vi "Ordering System.vi"() -> ()   [LabVIEW 2022 SP3]
panel:
  out "Waiting time":i32
  in  "Place your order":bool
  out "Discount %":string
  out "Discounted Bill":dbl
  out "Bill":dbl
  out "Price 5":dbl
  in  "Quantity":dbl=1.0 min=1.0 max=10.0 step=1.0
  in  "Item #1 5":bool
  out "Price 4":dbl
  in  "Quantity":dbl=1.0 min=1.0 max=10.0 step=1.0
  in  "Item #4":bool
  out "Price 3":dbl
  in  "Quantity":dbl=1.0 min=1.0 max=10.0 step=1.0
  in  "Item #3":bool
  out "Price 2":dbl
  in  "Quantity":dbl=1.0 min=1.0 max=10.0 step=1.0
  in  "Item #2":bool
  out "Price":dbl
  in  "Quantity":dbl=1.0 min=1.0 max=10.0 step=1.0
  in  "Item #1":bool
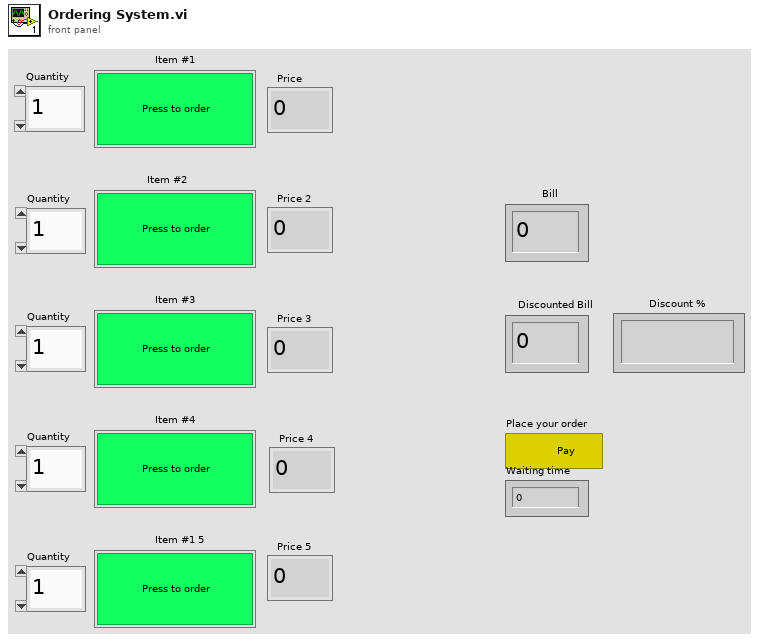
[diagram p1: front panel]
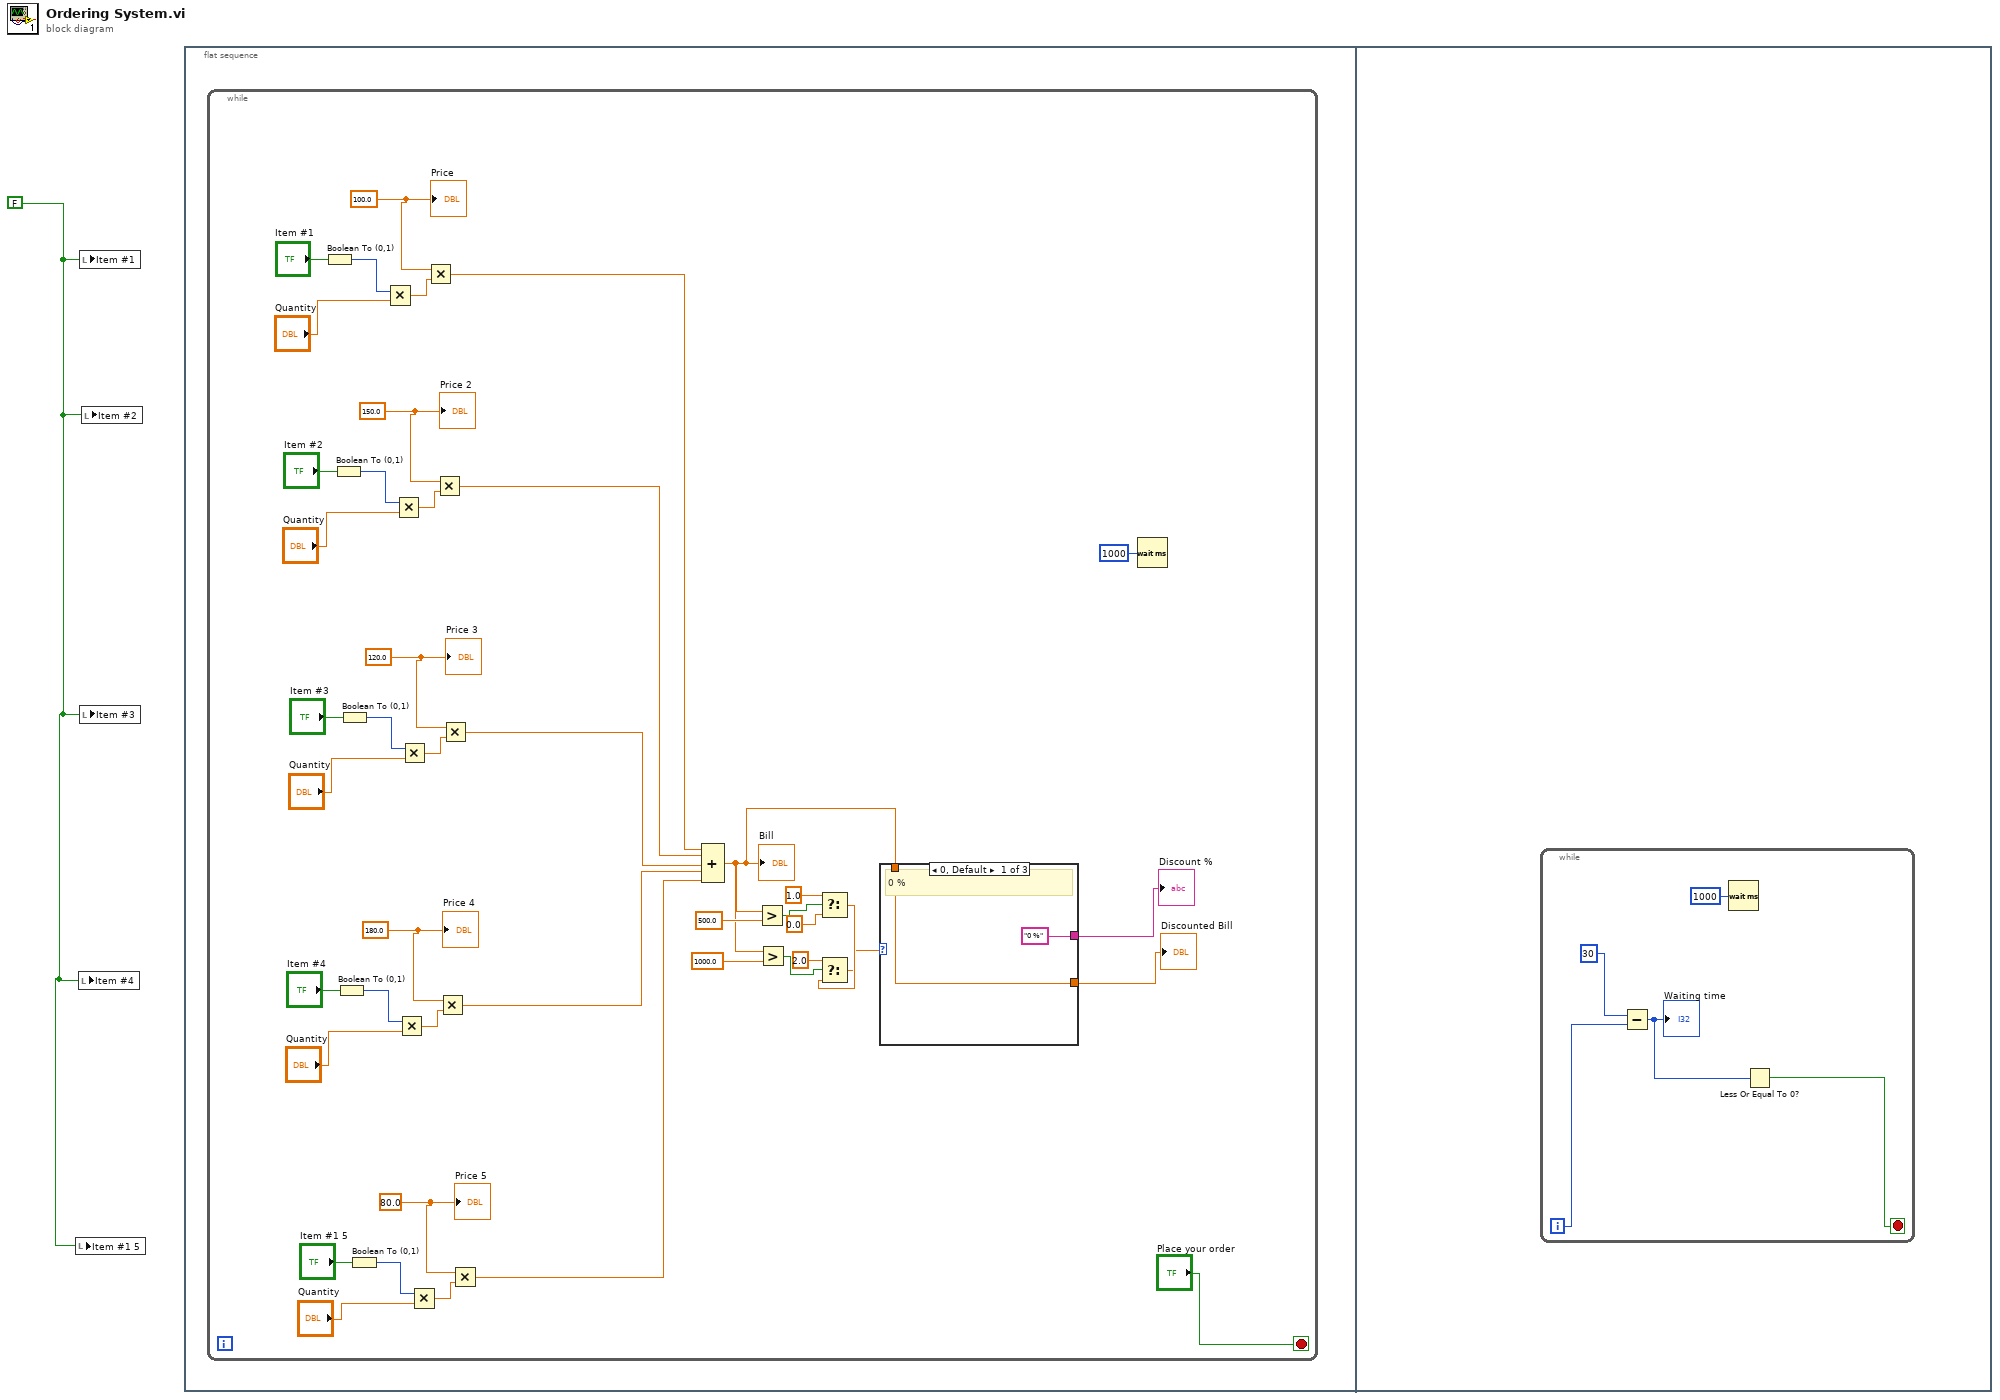
[diagram p0: block diagram]
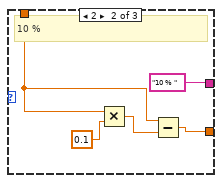
[diagram p2: hidden frame]
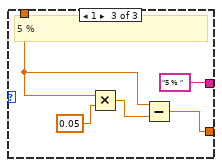
[diagram p3: hidden frame]
diagram:
  w1 = FALSE ("Item #1")
  n1 = local write "Item #1 5"(w1) -> ()
  n2 = local write "Item #4"(w1) -> ()
  n3 = local write "Item #1"(w1) -> ()
  n4 = local write "Item #3"(w1) -> ()
  n5 = local write "Item #2"(w1) -> ()
  n6 = flat-sequence {
    frame #0 {
      n7 = while {
        stop <- "Place your order" stop-if-true
        w21 = 80.0 ("Price")
        w26 = 180.0 ("Price")
        w31 = 120.0 ("Price")
        w36 = 150.0 ("Price")
        w41 = 100.0 ("Price")
        n8 = Boolean To (0,1)(Boolean="Item #1") -> (0, 1=w44:i16)
        n9 = Boolean To (0,1)(Boolean="Item #2") -> (0, 1=w39:i16)
        n10 = Boolean To (0,1)(Boolean="Item #4") -> (0, 1=w29:i16)
        n11 = Boolean To (0,1)(Boolean="Item #3") -> (0, 1=w34:i16)
        n12 = Boolean To (0,1)(Boolean="Item #1 5") -> (0, 1=w24:i16)
        n13 = Multiply(x=w44, y="Quantity") -> (x*y=w42:dbl)
        n14 = Multiply(x=w39, y="Quantity") -> (x*y=w37:dbl)
        n15 = Multiply(x=w29, y="Quantity") -> (x*y=w27:dbl)
        n16 = Multiply(x=w34, y="Quantity") -> (x*y=w32:dbl)
        n17 = Multiply(x=w24, y="Quantity") -> (x*y=w22:dbl)
        n18 = Multiply(x=w41, y=w42) -> (x*y=w20:dbl)
        n19 = Multiply(x=w36, y=w37) -> (x*y=w19:dbl)
        n20 = Multiply(x=w26, y=w27) -> (x*y=w17:dbl)
        n21 = Multiply(x=w31, y=w32) -> (x*y=w18:dbl)
        n22 = Multiply(x=w21, y=w22) -> (x*y=w16:dbl)
        n23 = Compound Arithmetic op=ADD(w20, w19, w18, w17, w16) -> (w7:dbl)
        "Bill" <- w7
        n24 = Greater?(x=w7, y=500.0) -> (0:w11:bool)
        n25 = Greater?(x=w7, y=1000.0) -> (0:w10:bool)
        n26 = Select(t=1.0 ("s? t:f"), s=w11, f=0.0 ("s? t:f")) -> (s? t:f=w9:dbl)
        n27 = Select(t=2.0 ("s? t:f"), s=w10, f=w9) -> (s? t:f=w6:dbl)
        n28 = case shown="0, Default" w6 {
          tunnel: [w47 w49 w54] -> w8
          tunnel: w7 -> [w47 w50 w55]
          tunnel: ["0 %" ("Discount %") "10 % " ("Discount %") "5 % " ("Discount %")] -> w5
          frame 0, Default {
            # "0 %"
          }
          frame 2 {
            # "10 %"
            n29 = Multiply(x=w50, y=0.1 ("x*y")) -> (x*y=w52:dbl)
            n30 = Subtract(x=w50, y=w52) -> (x-y=w49:dbl)
          }
          frame 1 {
            # "5 %"
            n31 = Multiply(x=w55, y=0.05 ("x*y")) -> (x*y=w56:dbl)
            n32 = Subtract(x=w55, y=w56) -> (x-y=w54:dbl)
          }
        }
        "Discounted Bill" <- w8
        "Discount %" <- w5
        n33 = Wait (ms)(milliseconds to wait=u32 1000) -> ()  [unwired: 1 out]
        "Price" <- w41
        "Price 2" <- w36
        "Price 3" <- w31
        "Price 4" <- w26
        "Price 5" <- w21
      }
    }
    frame #1 {
      n34 = while {
        i -> [w62]
        stop <- w59 stop-if-true
        n35 = Subtract(x=30, y=w62) -> (x-y=w60:i32)
        "Waiting time" <- w60
        n36 = Wait (ms)(milliseconds to wait=u32 1000) -> ()  [unwired: 1 out]
        n37 = Less Or Equal To 0?(x=w60) -> (x <= 0?=w59:bool)
      }
    }
  }
